vi "Execute.vi"(8 "error in (no error)":errorcluster, 11 "Pressure Calibration Command in":refnum<class "Pressure Calibration Command.lvclass">) -> (0 "error out":errorcluster, 3 "Pressure Calibration Command out":refnum<class "Pressure Calibration Command.lvclass">)   [LabVIEW 2014, in "Pressure Calibration Command.lvclass"]
uses:
  Pressure Calibration Command.lvclass
  Reusable/Commands/Command.lvclass
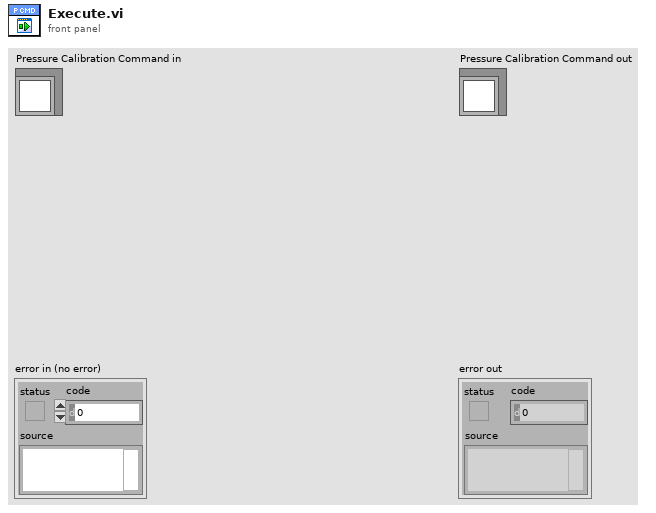
[diagram p1: front panel]
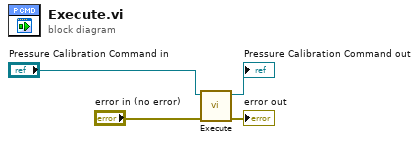
[diagram p0: block diagram]
diagram:
  n1 = call-parent "Execute.vi"("error in"="error in (no error)", "Instrument In"="Pressure Calibration Command in") -> ("error out"=→"error out":errorcluster, "Instrument Out"=→"Pressure Calibration Command out":refnum<class>)  [unwired: 8 in]
